vi "sequenceTEster.vi"() -> ()   [LabVIEW 2019]
uses:
  <vilib>/numeric/Random Number (Range) I64.vi
  <vilib>/numeric/sub_Random U32.vi
  LED Class/LED.lvclass
panel:
  out "Numeric":i32
  in  "stop":bool
  out "Yellow":bool
  out "Green":bool
  out "Red":bool
  out "Blue":bool
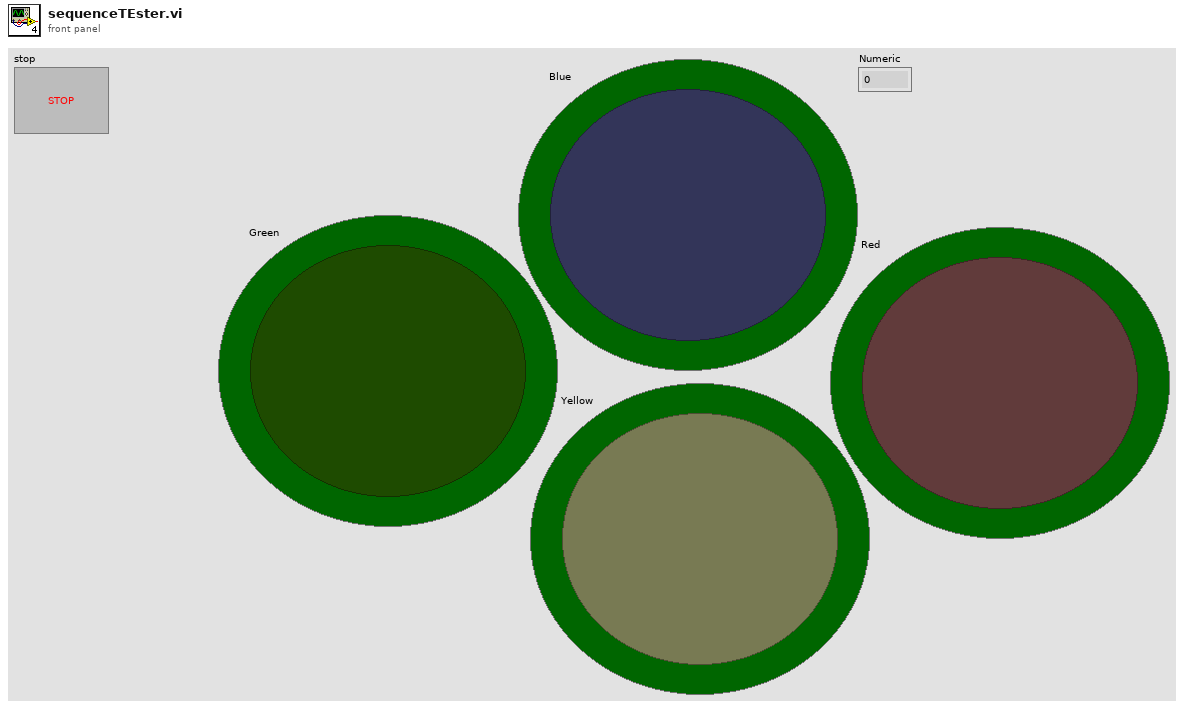
[diagram p1: front panel]
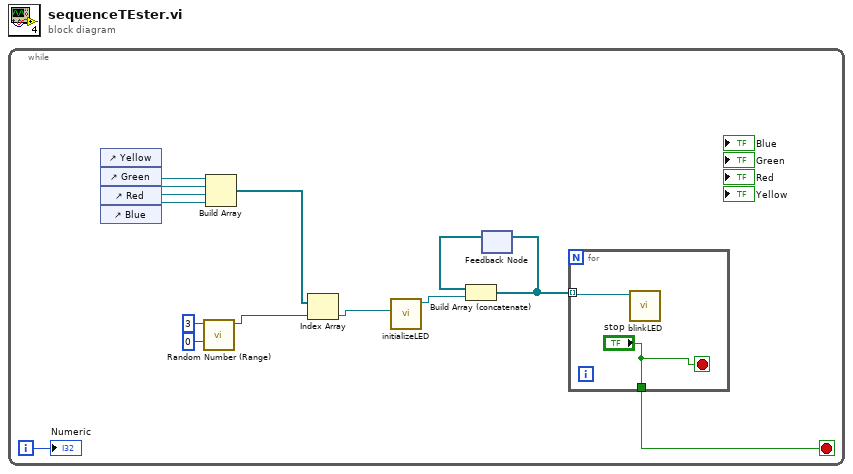
[diagram p0: block diagram]
diagram:
  n1 = while {
    i -> [w2]
    stop <- w1 stop-if-true
    n2 = control-ref of="Yellow"() -> (w12:refnum<vi>)
    n3 = control-ref of="Green"() -> (w11:refnum<vi>)
    n4 = control-ref of="Red"() -> (w10:refnum<vi>)
    n5 = control-ref of="Blue"() -> (w9:refnum<vi>)
    n6 = call-poly <vilib>:"Random Number (Range).vi"("lower bound (-100)"=i64 0, "upper bound (100)"=i64 3) -> ("number"=w7:i64)  [unwired: 9 in]
    n7 = Build Array(w12, w11, w10, w9) -> (w8:refnum<vi>[])
    n8 = Index Array(array=w8, index=w7) -> (element=w4:refnum<vi>)
    n9 = call "initializeLED.vi"("LED Refnum"=w4) -> ("LED out"=w14:refnum<class "LED.lvclass">)  [unwired: 9 in, 1 out]
    n10 = feedback #1() -> (w13:refnum<class "LED.lvclass">[])  [unwired: 1 in]
    n11 = Build Array (concatenate)(w13, w14) -> (w3:refnum<class "LED.lvclass">[])
    n12 = feedback-in #1(w3) -> ()
    n13 = for {
      tunnel: w3 -> [w16] mode=indexing
      tunnel: ["stop"] -> w1
      stop <- "stop" stop-if-true
      n14 = call "blinkLED.vi"("LED in"=w16) -> ()  [unwired: 9 in, 2 out]
    }
    "Numeric" <- w2
  }
